vi "Left Motor Loops (SubVI).vi"   [LabVIEW 2015]
uses:
  <vilib>/Platform/TimedLoop/XDataNode/timing_clust.ctl
  <vilib>/Platform/TimedLoop/XDataNode/nitl_modes.ctl
  <vilib>/Platform/TimedLoop/XDataNode/wakeup.ctl
  Left Variables.vi
  <vilib>/Utility/error.llb/Error Cluster From Error Code.vi
  <vilib>/myRIO/Common/Instrument Driver Framework/myRIO v1.0/DIO/vis/myRIO v1.0 Write DIO.vi
  <vilib>/platform/TimedLoop/XDataNode/XDataNode.xnode
  <vilib>/myRIO/Instrument Drivers/Onboard IO/DIO/DIO.lvlib
  <vilib>/Platform/TimedLoop/XDataNode/XDNodeRunTimeDep.lvlib
types:
  T1 = typedef "DIO.lvlib/DIO Reference.ctl" = cluster{"myRIO Reference":T2, "DIO Channels List":T6}
  T2 = typedef "myRIO Generic Hardware Reference.ctl" = cluster{"myRIO Model":T3, "myRIO Hardware Reference":T4}
  T3 = typedef "Hardware Version Enum.ctl" = enum16{"Unknown", "myRIO-1900", "myRIO-1950", "roboRIO"}
  T4 = typedef "myRIO v1.0 Reference.ctl" = cluster{"Generic FPGA Reference":T5, "Allow multiple opens":bool}
  T5 = typedef "Generic FPGA Reference.ctl" = refnum<k20>
  T6 = typedef "DIO Channels List.ctl" = T7[]
  T7 = typedef "DIO Channels Enum.ctl" = enum16{"Not Connected", "C/DIO0", "C/DIO1", "C/DIO2", "C/DIO3", "C/DIO4", "C/DIO5", "C/DIO6", "C/DIO7", "A/DIO0", "A/DIO1", "A/DIO2", "A/DIO3", "A/DIO4", "A/DIO5", "A/DIO6", "A/DIO7", "A/DIO8", "A/DIO9", "A/DIO10", "A/DIO11", "A/DIO12", "A/DIO13", "A/DIO14", "A/DIO15", "B/DIO0", "B/DIO1", "B/DIO2", "B/DIO3", "B/DIO4", "B/DIO5", "B/DIO6", "B/DIO7", "B/DIO8", "B/DIO9", "B/DIO10", "B/DIO11", "B/DIO12", "B/DIO13", "B/DIO14", "B/DIO15", "LED0", "LED1", "LED2", "LED3", "Button0", "DIO/DIO0", "DIO/DIO1", "DIO/DIO2", "DIO/DIO3", "DIO/DIO4", "DIO/DIO5", "DIO/DIO6", "DIO/DIO7", "DIO/DIO8", "DIO/DIO9", "SPI/CS0", "SPI/CS1", "SPI/CS2", "SPI/CS3", "LED RADIO (Green)", "LED RADIO (Red)", "LED COMM (Green)", "LED COMM (Red)", "LED MODE (Green)", "LED MODE (Red)"}
  T8 = typedef "XDNodeRunTimeDep.lvlib/timing_clust.ctl" = cluster{"Expected End [f-1]":u64, "Actual End [f-1]":u64, "Finished Late? [f-1]":bool, "Expected End [i-1]":u64, "Actual End [i-1]":u64, "Finished Late? [i-1]":bool, "Expected Start [i]":u64, "Actual Start [i]":u64, "Expected Start [f]":u64, "Actual Start [f]":u64, "Source Name":string, "Structure Name":string, "Period":i64, "Deadline":i64, "Offset":i64, "Start":i64, "Priority":i32, "Timeout":i32, "Mode":T9, "Wakeup Reason":T10, "Error":errorcluster, "Source Type":string, "Secondary Source Type":string, "Global End Time":u64, "Global Start Time":u64, "Frame Duration":u64, "Iteration Duration":u64, "Assigned CPU":i32, "I/O Scan Engine Mode":u32}
  T9 = typedef "XDNodeRunTimeDep.lvlib/nitl_modes.ctl" = enum32{"No Change", "Process missed periods, maintain original phase", "Discard missed periods, maintain original phase", "Process missed periods, ignore original phase", "Discard missed periods, ignore original phase"}
  T10 = typedef "XDNodeRunTimeDep.lvlib/wakeup.ctl" = enum32{"Normal", "Aborted", "Asynchronous wakeup", "Timing source error", "Timed loop error", "Timeout"}
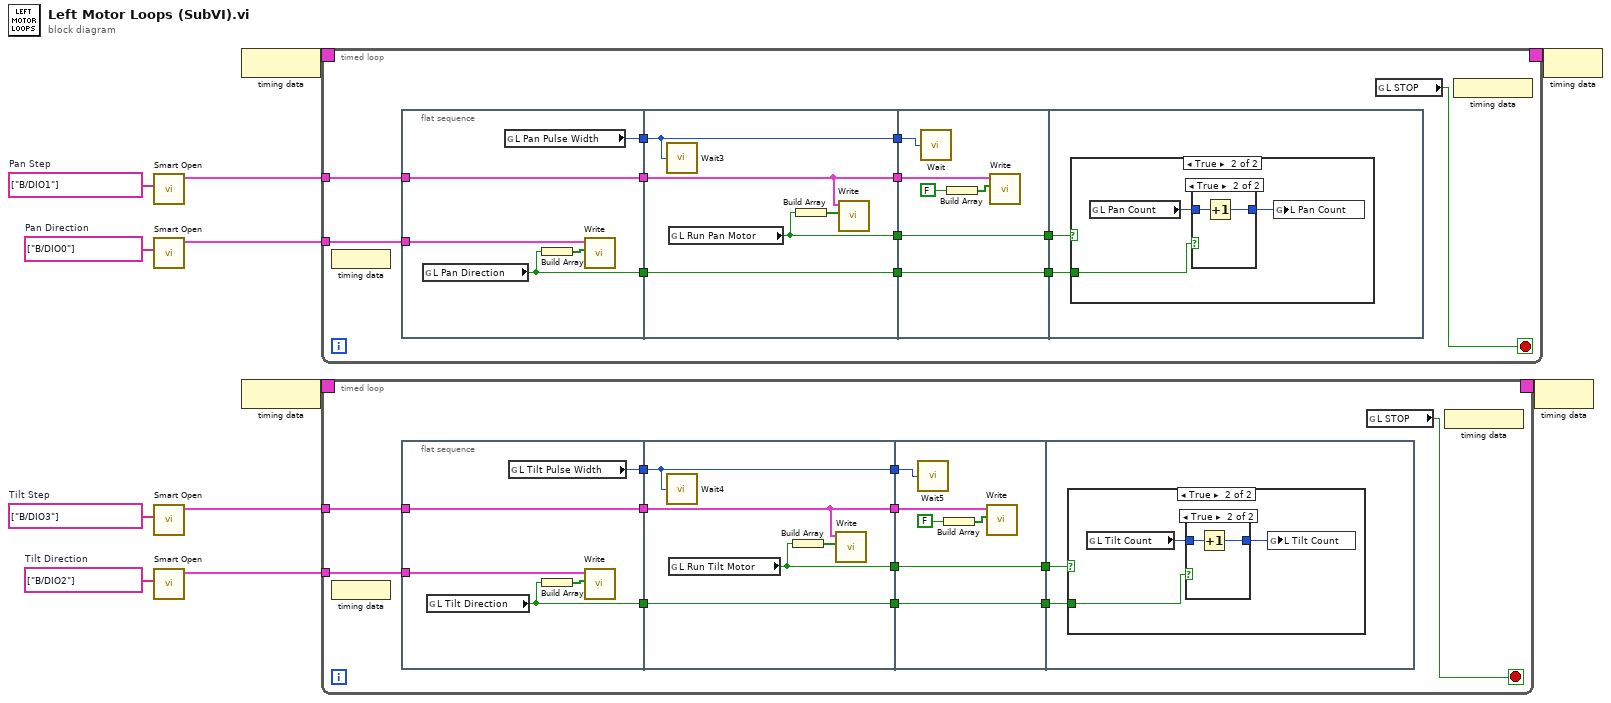
[diagram p0: block diagram]
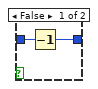
[diagram p3: hidden frame]
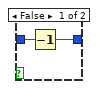
[diagram p5: hidden frame]
diagram:
  w2 = tag[] ["B/DIO2"]  # Tilt Direction
  w4 = tag[] ["B/DIO3"]  # Tilt Step
  w8 = tag[] ["B/DIO0"]  # Pan Direction
  w10 = tag[] ["B/DIO1"]  # Pan Step
  n1 = call <vilib>:"Smart Open.vi"("Channel Names"=w10) -> ("DIO Ref Out"=w9:T1)  [unwired: 9 in, 1 out]
  n2 = call <vilib>:"Smart Open.vi"("Channel Names"=w8) -> ("DIO Ref Out"=w7:T1)  [unwired: 9 in, 1 out]
  n3 = call <vilib>:"Smart Open.vi"("Channel Names"=w4) -> ("DIO Ref Out"=w3:T1)  [unwired: 9 in, 1 out]
  n4 = call <vilib>:"Smart Open.vi"("Channel Names"=w2) -> ("DIO Ref Out"=w1:T1)  [unwired: 9 in, 1 out]
  n5 = node-c288() -> (w12:T8)
  n6 = node-c288() -> (w6:T8)
  n7 = timed-loop {
    timing: w12 -> [_]
    timing-out: [_] -> w11
    tunnel: w9 -> [w19]
    tunnel: w7 -> [w18]
    stop <- w17 stop-if-true
    n8 = node-c288() -> ()  [unwired: 1 in]
    n9 = flat-sequence {
      tunnel: [w27] -> w24
      tunnel: [w29] -> w20
      tunnel: w19 -> [w29]
      tunnel: w18 -> [w28]
      tunnel: [w25] -> w16
      tunnel: [w34] -> w23
      tunnel: w24 -> [w34]
      tunnel: [w33] -> w21
      tunnel: w20 -> [w33]
      tunnel: w16 -> [w31]
      tunnel: [w31] -> w15
      tunnel: [w30] -> w13
      tunnel: [w40] -> w22
      tunnel: w23 -> [w40]
      tunnel: w21 -> [w37]
      tunnel: w15 -> [w36]
      tunnel: [w35] -> w14
      tunnel: w13 -> [w35]
      tunnel: w22 -> [w42]
      tunnel: w14 -> [w41]
      frame #0 {
        n10 = global read "Left Variables.vi" "L Pan Direction"() -> (w27:bool)
        n11 = global read "Left Variables.vi" "L Pan Pulse Width"() -> (w25:u32)
        n12 = Build Array(w27) -> (w26:bool[])
        n13 = call <vilib>:"Write.vi"("Values"=w26, "DIO Ref In"=w28) -> ()  [unwired: 7 in, 2 out]
      }
      frame #1 {
        n14 = call "Wait3"("Count(uSec)"=w31) -> ()  [unwired: 1 out]
        n15 = global read "Left Variables.vi" "L Run Pan Motor"() -> (w30:bool)
        n16 = Build Array(w30) -> (w32:bool[])
        n17 = call <vilib>:"Write.vi"("Values"=w32, "DIO Ref In"=w33) -> ()  [unwired: 7 in, 2 out]
      }
      frame #2 {
        n18 = call "Wait"("Count(uSec)"=w36) -> ()  [unwired: 1 out]
        n19 = Build Array(FALSE ("B/DIO1 (Pin 13)")) -> (w39:bool[])
        n20 = call <vilib>:"Write.vi"("Values"=w39, "DIO Ref In"=w37) -> ()  [unwired: 7 in, 2 out]
      }
      frame #3 {
        n21 = case shown="True" w41 {
          tunnel: w42 -> [_ w45]
          frame False {
          }
          frame True {
            n22 = global read "Left Variables.vi" "L Pan Count"() -> (w44:i32)
            n23 = case shown="True" w45 {
              tunnel: [w47 w49] -> w43
              tunnel: w44 -> [w46 w48]
              frame False {
                n24 = Decrement(x=w46) -> (x-1=w47:i32)
              }
              frame True {
                n25 = Increment(x=w48) -> (x+1=w49:i32)
              }
            }
            n26 = global write "Left Variables.vi" "L Pan Count"(w43) -> ()
          }
        }
      }
    }
    n27 = global read "Left Variables.vi" "L STOP"() -> (w17:bool)
    n28 = node-c288() -> ()  [unwired: 1 out]
  }
  n29 = timed-loop {
    timing: w6 -> [_]
    timing-out: [_] -> w5
    tunnel: w3 -> [w58]
    tunnel: w1 -> [w57]
    stop <- w56 stop-if-true
    n30 = node-c288() -> ()  [unwired: 1 in]
    n31 = flat-sequence {
      tunnel: [w66] -> w63
      tunnel: [w68] -> w59
      tunnel: w58 -> [w68]
      tunnel: w57 -> [w67]
      tunnel: [w64] -> w55
      tunnel: [w73] -> w62
      tunnel: w63 -> [w73]
      tunnel: [w72] -> w60
      tunnel: w59 -> [w72]
      tunnel: w55 -> [w70]
      tunnel: [w70] -> w54
      tunnel: [w69] -> w52
      tunnel: [w79] -> w61
      tunnel: w62 -> [w79]
      tunnel: w60 -> [w76]
      tunnel: w54 -> [w75]
      tunnel: [w74] -> w53
      tunnel: w52 -> [w74]
      tunnel: w61 -> [w81]
      tunnel: w53 -> [w80]
      frame #0 {
        n32 = global read "Left Variables.vi" "L Tilt Direction"() -> (w66:bool)
        n33 = global read "Left Variables.vi" "L Tilt Pulse Width"() -> (w64:u32)
        n34 = Build Array(w66) -> (w65:bool[])
        n35 = call <vilib>:"Write.vi"("Values"=w65, "DIO Ref In"=w67) -> ()  [unwired: 7 in, 2 out]
      }
      frame #1 {
        n36 = call "Wait4"("Count(uSec)"=w70) -> ()  [unwired: 1 out]
        n37 = global read "Left Variables.vi" "L Run Tilt Motor"() -> (w69:bool)
        n38 = Build Array(w69) -> (w71:bool[])
        n39 = call <vilib>:"Write.vi"("Values"=w71, "DIO Ref In"=w72) -> ()  [unwired: 7 in, 2 out]
      }
      frame #2 {
        n40 = call "Wait5"("Count(uSec)"=w75) -> ()  [unwired: 1 out]
        n41 = Build Array(FALSE ("B/DIO1 (Pin 13)")) -> (w78:bool[])
        n42 = call <vilib>:"Write.vi"("Values"=w78, "DIO Ref In"=w76) -> ()  [unwired: 7 in, 2 out]
      }
      frame #3 {
        n43 = case shown="True" w80 {
          tunnel: w81 -> [_ w84]
          frame False {
          }
          frame True {
            n44 = global read "Left Variables.vi" "L Tilt Count"() -> (w83:i32)
            n45 = case shown="True" w84 {
              tunnel: [w86 w88] -> w82
              tunnel: w83 -> [w85 w87]
              frame False {
                n46 = Decrement(x=w85) -> (x-1=w86:i32)
              }
              frame True {
                n47 = Increment(x=w87) -> (x+1=w88:i32)
              }
            }
            n48 = global write "Left Variables.vi" "L Tilt Count"(w82) -> ()
          }
        }
      }
    }
    n49 = global read "Left Variables.vi" "L STOP"() -> (w56:bool)
    n50 = node-c288() -> ()  [unwired: 1 out]
  }
  n51 = node-c288(w5) -> ()
  n52 = node-c288(w11) -> ()
